vi "RT_Main.vi"() -> ()   [LabVIEW 2018]
uses:
  <vilib>/Utility/RT CPU Load.ctl
  <vilib>/Platform/TimedLoop/XDataNode/timing_clust.ctl
  <vilib>/Platform/TimedLoop/XDataNode/nitl_modes.ctl
  <vilib>/Platform/TimedLoop/XDataNode/wakeup.ctl
  <vilib>/platform/TimedLoop/XDataNode/XDataNode.xnode
  <vilib>/Platform/TimedLoop/XDataNode/XDNodeRunTimeDep.lvlib
  <vilib>/NI_Real-Time Target Support.lvlib
panel:
  out "CPU loads":T1[](array[typedef]) {"ISR (%)" format="%#.2f"; "Idle (%)" format="%#.2f"; "Background (%)" format="%#.2f"; "Normal (%)" format="%#.2f"; "Above Normal (%)" format="%#.2f"; "High (%)" format="%#.2g"; "Timed Structures (%)" format="%#.2g"; "Time Critical (%)" format="%#.2g"; "Total (%)" format="%#.2g"}
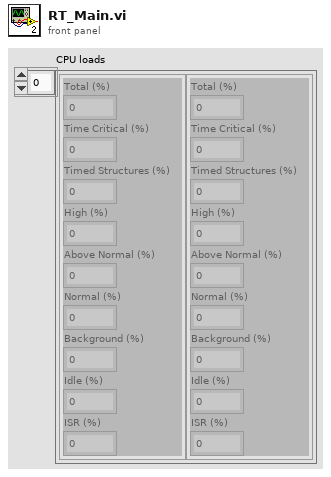
[diagram p1: front panel]
types:
  T1 = typedef "NI_Real-Time Target Support.lvlib/RT CPU Load.ctl" = cluster{"Total (%)":dbl, "Time Critical (%)":dbl, "Timed Structures (%)":dbl, "High (%)":dbl, "Above Normal (%)":dbl, "Normal (%)":dbl, "Background (%)":dbl, "Idle (%)":dbl, "ISR (%)":dbl}
  T2 = typedef "RT_Main Data.ctl" = cluster{"FPGA VI Reference":T3, "Listener ID":refnum<k5>, "Request Queue":refnum<queue>}
  T3 = typedef "RT_FPGA VI Reference.ctl" = refnum<k20>
  T4 = typedef "XDNodeRunTimeDep.lvlib/timing_clust.ctl" = cluster{"Expected End [f-1]":u64, "Actual End [f-1]":u64, "Finished Late? [f-1]":bool, "Expected End [i-1]":u64, "Actual End [i-1]":u64, "Finished Late? [i-1]":bool, "Expected Start [i]":u64, "Actual Start [i]":u64, "Expected Start [f]":u64, "Actual Start [f]":u64, "Source Name":string, "Structure Name":string, "Period":i64, "Deadline":i64, "Offset":i64, "Start":i64, "Priority":i32, "Timeout":i32, "Mode":T5, "Wakeup Reason":T6, "Error":errorcluster, "Source Type":string, "Secondary Source Type":string, "Global End Time":u64, "Global Start Time":u64, "Frame Duration":u64, "Iteration Duration":u64, "Assigned CPU":i32, "I/O Scan Engine Mode":u32}
  T5 = typedef "XDNodeRunTimeDep.lvlib/nitl_modes.ctl" = enum32{"No Change", "Process missed periods, maintain original phase", "Discard missed periods, maintain original phase", "Process missed periods, ignore original phase", "Discard missed periods, ignore original phase"}
  T6 = typedef "XDNodeRunTimeDep.lvlib/wakeup.ctl" = enum32{"Normal", "Aborted", "Asynchronous wakeup", "Timing source error", "Timed loop error", "Timeout"}
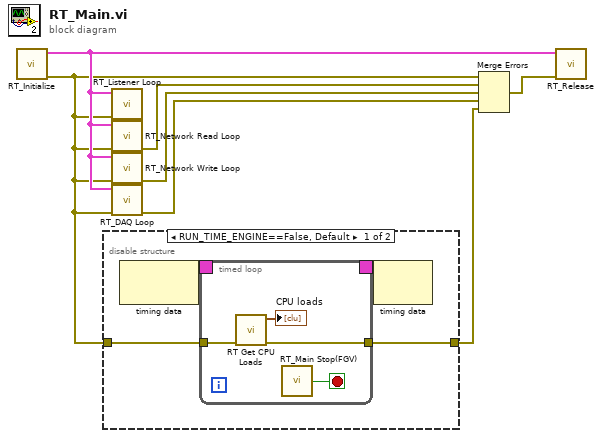
[diagram p0: block diagram]
diagram:
  n1 = call "RT_Initialize.vi"() -> ("error out"=w2:errorcluster, "Main Data"=w7:T2)  [unwired: 10 in]
  n2 = disable-structure shown="RUN_TIME_ENGINE==False, Default" {
    disable-tunnel: w2 -> [w9 w20]
    disable-tunnel: [w8 w20] -> w1
    frame condition #0 (active) {
      n3 = node-c288() -> (w11:T4)  [unwired: 1 in]
      n4 = timed-loop {
        timing: w11 -> [_]
        timing-out: [_] -> w10
        tunnel: w9 -> [w15]
        tunnel: [w12] -> w8
        stop <- w13 stop-if-true
        n5 = call <vilib>:"RT Get CPU Loads.vi"("error in (no error)"=w15) -> ("error out"=w12:errorcluster, "CPU loads"=→"CPU loads":T1[])  [unwired: 9 in]
        n6 = call "RT_Main Stop(FGV).vi"() -> ("Stop Out"=w13:bool)  [unwired: 4 in]
      }
      n7 = node-c288(w10) -> ()  [unwired: 1 out]
    }
    frame condition #1 {
    }
  }
  n8 = call "RT_Listener Loop.vi"("error in"=w2, "Main Data"=w7) -> ()  [unwired: 10 in]
  n9 = call "RT_Network Read Loop.vi"("error in"=w2, "Main Data"=w7) -> ("error out"=w6:errorcluster)  [unwired: 9 in]
  n10 = call "RT_Network Write Loop.vi"("error in"=w2, "Main Data"=w7) -> ("error out"=w5:errorcluster)  [unwired: 9 in]
  n11 = call "RT_DAQ Loop.vi"("error in"=w2, "Main Data"=w7) -> ("error out"=w4:errorcluster)  [unwired: 9 in]
  n12 = Merge Errors(w2, w6, w5, w4, w1) -> (w3:errorcluster)
  n13 = call "RT_Release.vi"("error in"=w3, "Main Data"=w7) -> ()  [unwired: 9 in, 1 out]
